vi "Measure.vi"() -> ()   [LabVIEW 2013]
uses:
  <vilib>/Utility/error.llb/DialogType.ctl
panel:
  in  "errorOutt":errorcluster
  in  "m1":string=" INSTRUCTIONS:\r\rNormal Use:  When using subVIs that incorporate the error in/error out (or error I/O) structure, place this handler where you want to inform the user of an error, typically at the end of the I/O data path, as the last action of the program.  If the error in error? is ERROR, the handler creates a message describing the error and its source.  If the type of dialog = 1 (default), the message is displayed to the user, who can only acknowedge it.  If the type = 2, the user can acknowledge the message or abort execution; aborting a program with active I/O is not recommended.  If the type = 0, no message is displayed; this is used to process the error programmatically, and the error out cluster elements are wired to individual terminals for that reason.  \r\rOther Use:\n\r\nlocal testing.  To test the error code of a subVI or function that does not have the error I/O structure, you can wire its error code and a source string to the local error code and error source inputs.  If error in error? indicates no error and error code is not equal to 0, the local code and source are substituted for the error in values, and error? is set TRUE (ERROR)."
  in  "Error":bool
  in  "SetOutput":bool
  in  "NeedToSetOutput":bool
  out "Output":string
  out "SetCurrentStr":string
  out "SetVoltageStr":string
  in  "SetVoltage":dbl format="%#.3g"
  in  "SetCurrent":dbl
  in  "NeedToSetVoltage":bool
  in  "NeedToSetCurrent":bool
  in  "Active":bool
  out "connection ID":refnum<k5>
  in  "Connect":bool
  out "GetCurrent":string
  in  "Adress":string="172.16.21.19"
  out "GetVoltage":string
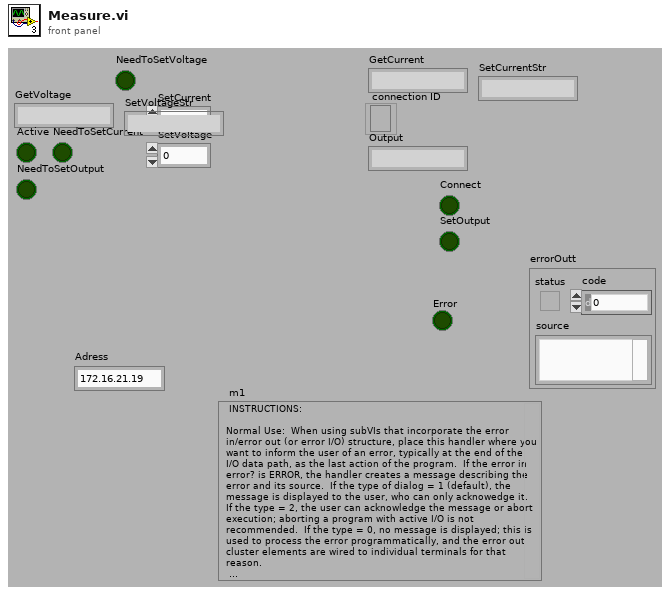
[diagram p1: front panel]
types:
  T1 = typedef "DialogType.ctl" = u16
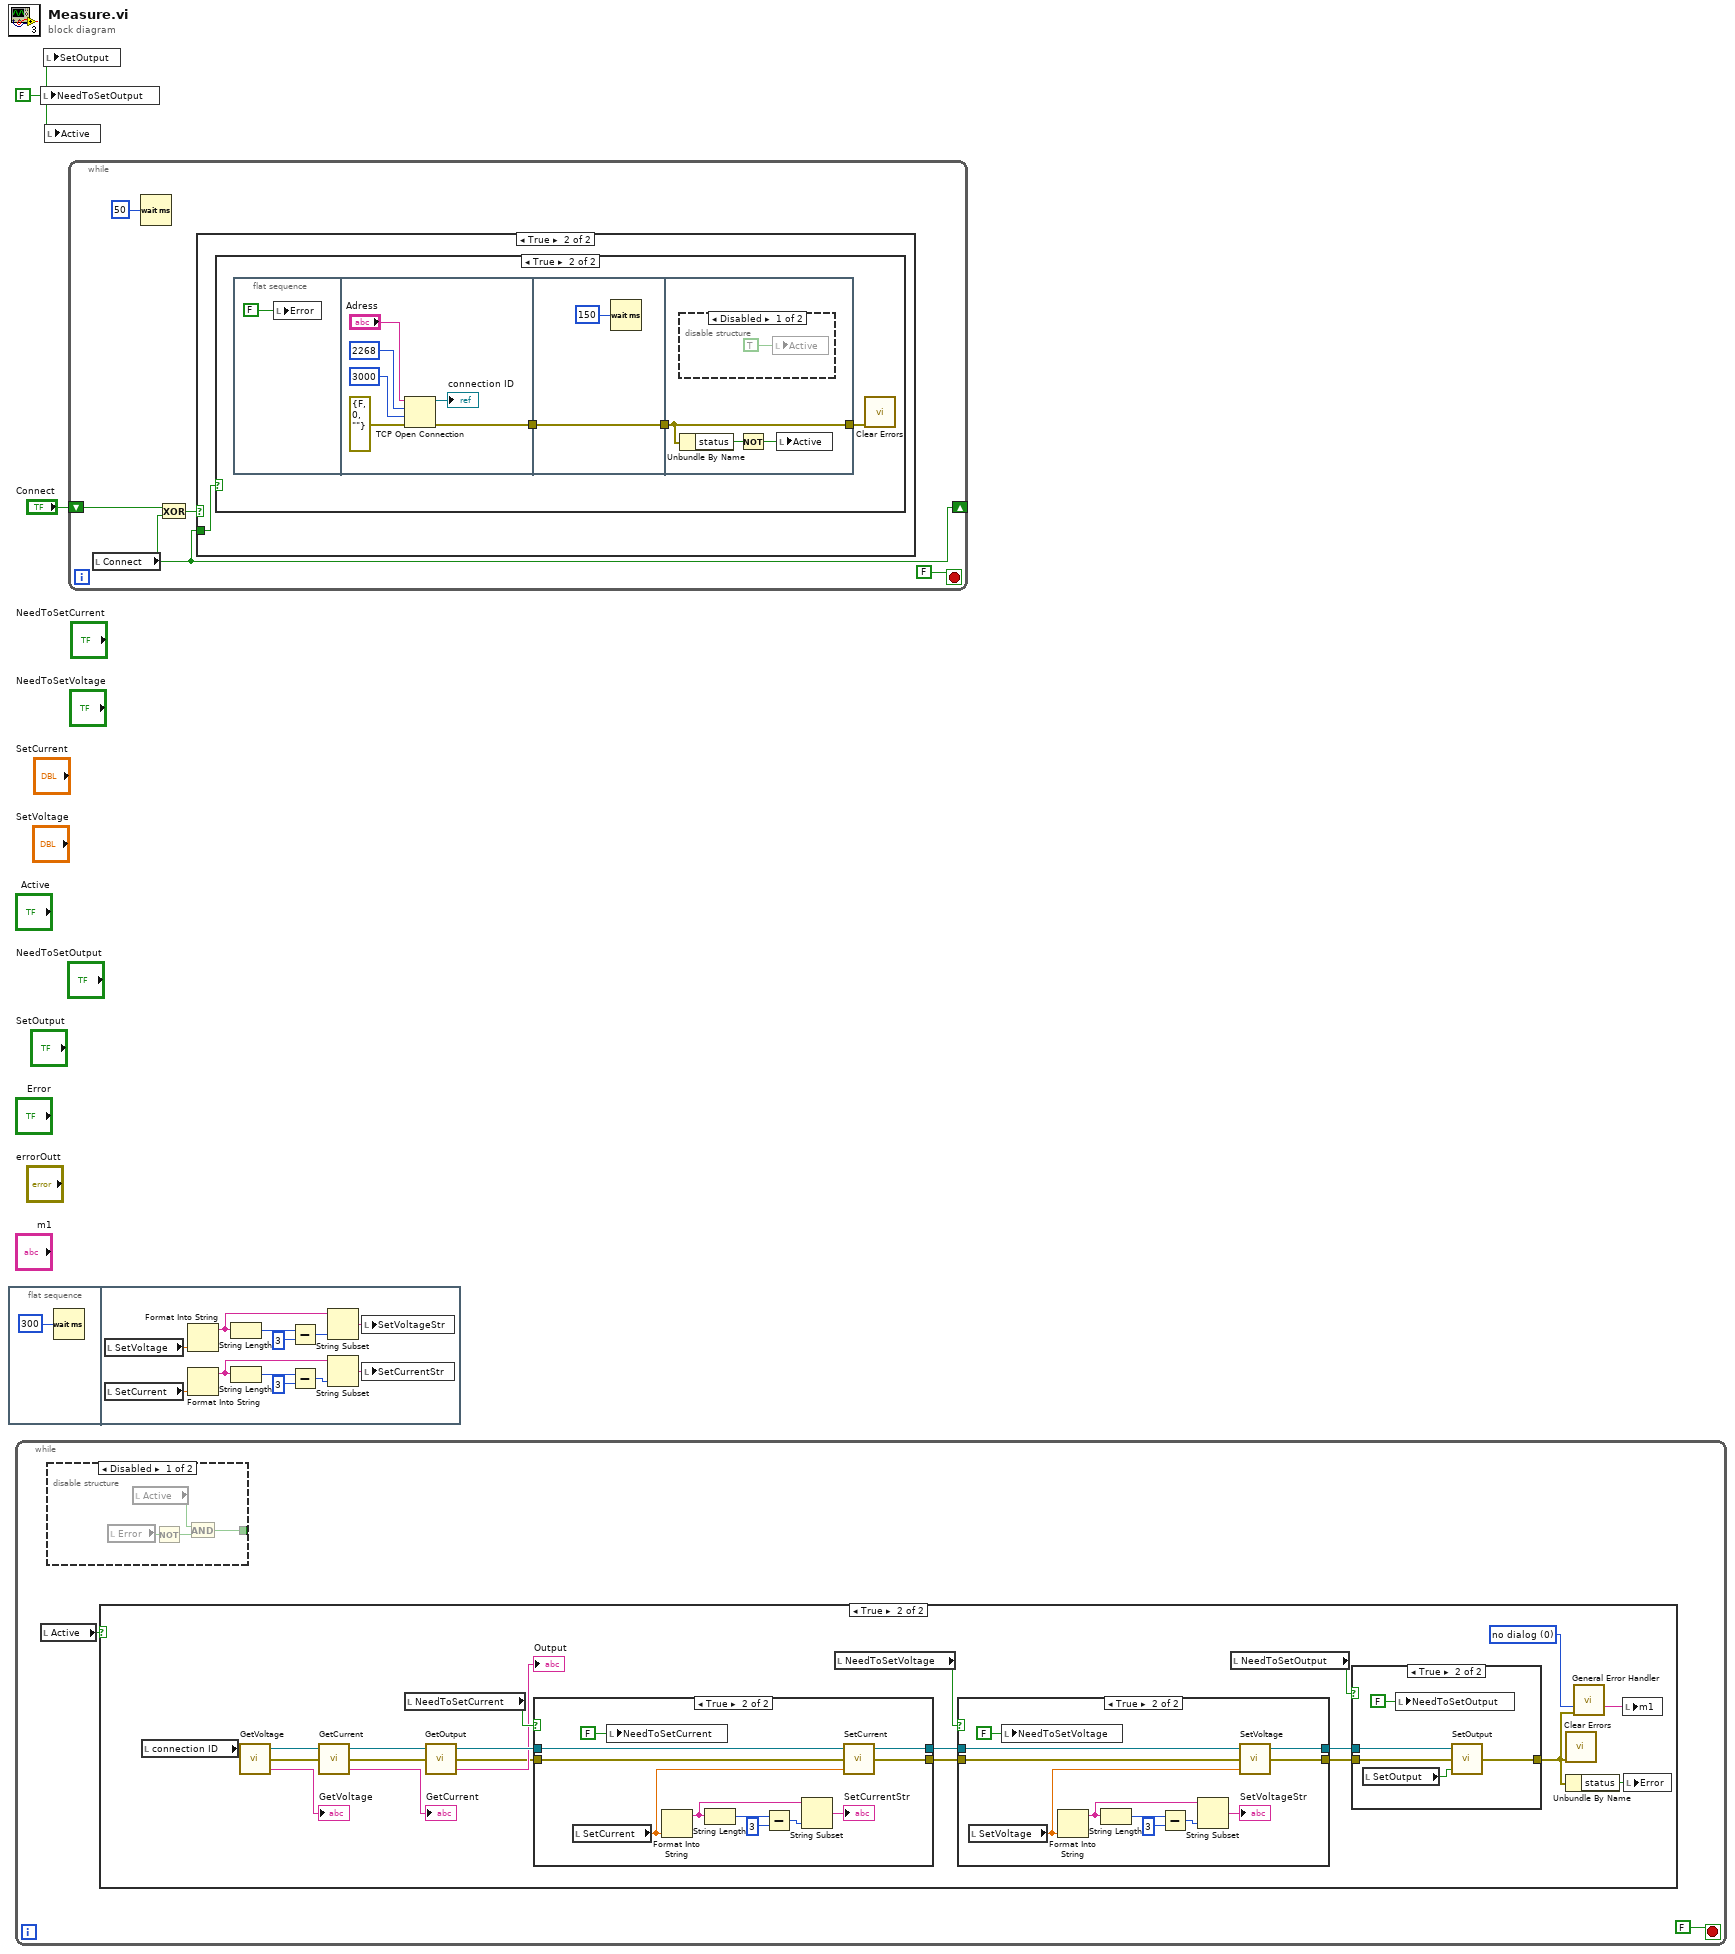
[diagram p0: block diagram]
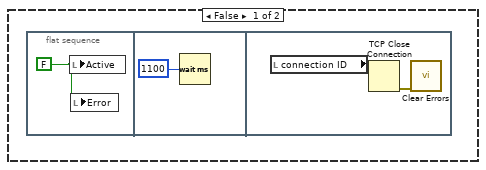
[diagram p8: hidden frame]
diagram:
  w1 = FALSE ("Active")
  n1 = flat-sequence {
    frame #0 {
      n2 = Wait (ms)(milliseconds to wait=u32 300 ("millisecond multiple")) -> ()  [unwired: 1 out]
    }
    frame #1 {
      n3 = local read "SetVoltage"() -> (w10:dbl)
      n4 = local read "SetCurrent"() -> (w11:dbl)
      n5 = Format Into String(w10) -> (resulting string=w6:string)  [unwired: 3 in, 1 out]
      n6 = Format Into String(w11) -> (resulting string=w15:string)  [unwired: 3 in, 1 out]
      n7 = String Length(string=w6) -> (length=w9:i32)
      n8 = String Length(string=w15) -> (length=w14:i32)
      n9 = Subtract(x=w9, y=3) -> (x-y=w7:i32)
      n10 = Subtract(x=w14, y=3) -> (x-y=w12:i32)
      n11 = String Subset(string=w6, length (rest)=w7) -> (substring=w5:string)  [unwired: 1 out]
      n12 = String Subset(string=w15, length (rest)=w12) -> (substring=w4:string)  [unwired: 1 out]
      n13 = local write "SetVoltageStr"(w5) -> ()
      n14 = local write "SetCurrentStr"(w4) -> ()
    }
  }
  n15 = while {
    stop <- FALSE stop-if-true
    n16 = local read "Active"() -> (w16:bool)
    n17 = disable-structure shown="Disabled" {
      disable-tunnel: [w18 _] -> _
      frame Disabled {
        n18 = local read "Error"() -> (w21:bool)
        n19 = local read "Active"() -> (w19:bool)
        n20 = Not(x=w21) -> (.not. x?=w20:bool)
        n21 = And(x=w19, y=w20) -> (x .and. y?=w18:bool)
      }
      frame Enabled {
      }
    }
    n22 = case shown="True" w16 {
      frame False {
      }
      frame True {
        w24 = T1 0 items=["no dialog", "OK message", "continue or stop message", "OK message + warnings", "continue/stop + warnings"] ("type of dialog (OK msg:1)")
        n23 = local read "connection ID"() -> (w39:refnum<k5>)
        n24 = call "GetVoltage.vi"("connection ID"=w39) -> ("Voltage"=→"GetVoltage":string, "error out"=w30:errorcluster, "connection ID out"=w41:refnum<k5>)  [unwired: 1 in, 1 out]
        n25 = call "GetCurrent.vi"("error in"=w30, "connection ID"=w41) -> ("Current"=→"GetCurrent":string, "error out"=w29:errorcluster, "connection ID out"=w35:refnum<k5>)  [unwired: 1 out]
        n26 = local read "NeedToSetCurrent"() -> (w36:bool)
        n27 = call "GetOutput.vi"("error in"=w29, "connection ID"=w35) -> ("Output"=→"Output":string, "error out"=w28:errorcluster, "connection ID out"=w34:refnum<k5>)  [unwired: 1 out]
        n28 = case shown="True" w36 {
          tunnel: w34 -> [w63 w74]
          tunnel: [w63 w73] -> w38
          tunnel: w28 -> [w62 w65]
          tunnel: [w62 w64] -> w27
          frame False {
          }
          frame True {
            n29 = local read "SetCurrent"() -> (w71:dbl)
            n30 = local write "NeedToSetCurrent"(FALSE ("NeedToSetCurrent")) -> ()
            n31 = Format Into String(w71) -> (resulting string=w66:string)  [unwired: 3 in, 1 out]
            n32 = String Length(string=w66) -> (length=w68:i32)
            n33 = Subtract(x=w68, y=3) -> (x-y=w70:i32)
            n34 = String Subset(string=w66, length (rest)=w70) -> (substring=→"SetCurrentStr":string)  [unwired: 1 out]
            n35 = call "SetCurrent.vi"("Current"=w71, "error in"=w65, "connection ID"=w74) -> ("error out"=w64:errorcluster, "connection ID out"=w73:refnum<k5>)  [unwired: 1 out]
          }
        }
        n36 = local read "NeedToSetVoltage"() -> (w37:bool)
        n37 = case shown="True" w37 {
          tunnel: w38 -> [w50 w61]
          tunnel: [w50 w53] -> w32
          tunnel: w27 -> [w49 w52]
          tunnel: [w49 w51] -> w26
          frame False {
          }
          frame True {
            n38 = local read "SetVoltage"() -> (w59:dbl)
            n39 = local write "NeedToSetVoltage"(FALSE ("NeedToSetVoltage")) -> ()
            n40 = Format Into String(w59) -> (resulting string=w55:string)  [unwired: 3 in, 1 out]
            n41 = String Length(string=w55) -> (length=w58:i32)
            n42 = Subtract(x=w58, y=3) -> (x-y=w56:i32)
            n43 = String Subset(string=w55, length (rest)=w56) -> (substring=→"SetVoltageStr":string)  [unwired: 1 out]
            n44 = call "SetVoltage.vi"("Voltage"=w59, "error in"=w52, "connection ID"=w61) -> ("error out"=w51:errorcluster, "connection ID out"=w53:refnum<k5>)  [unwired: 1 out]
          }
        }
        n45 = local read "NeedToSetOutput"() -> (w31:bool)
        n46 = case shown="True" w31 {
          tunnel: w32 -> [_ w46]
          tunnel: w26 -> [w43 w45]
          tunnel: [w43 w44] -> w22
          frame False {
          }
          frame True {
            n47 = local read "SetOutput"() -> (w47:bool)
            n48 = local write "NeedToSetOutput"(FALSE ("NeedToSetVoltage")) -> ()
            n49 = call "SetOutput.vi"("State"=w47, "error in"=w45, "connection ID"=w46) -> ("error out"=w44:errorcluster)  [unwired: 2 out]
          }
        }
        n50 = call <vilib>:"Clear Errors.vi"("error in (no error)"=w22) -> ()  [unwired: 7 out]
        n51 = Unbundle By Name(w22) -> ("status"=w25:bool)
        n52 = call <vilib>:"General Error Handler.vi"("type of dialog (OK msg:1)"=w24, "error in (no error)"=w22) -> ("message"=w23:string)  [unwired: 13 out]
        n53 = local write "m1"(w23) -> ()
        n54 = local write "Error"(w25) -> ()
      }
    }
  }
  n55 = local write "NeedToSetOutput"(w1) -> ()
  n56 = local write "SetOutput"(w1) -> ()
  n57 = local write "Active"(w1) -> ()
  n58 = while {
    shift-right: [w75] -> _
    shift-left: "Connect" -> [w76]
    stop <- FALSE stop-if-true
    n59 = local read "Connect"() -> (w75:bool)
    n60 = Wait (ms)(milliseconds to wait=u32 50 ("millisecond multiple")) -> ()  [unwired: 1 out]
    n61 = Exclusive Or(1:w75, 2:w76) -> (0:w77:bool)
    n62 = case shown="True" w77 {
      tunnel: w75 -> [_ w80]
      frame False {
      }
      frame True {
        n63 = case shown="True" w80 {
          frame False {
            n64 = flat-sequence {
              frame #0 {
                w81 = FALSE ("Active")
                n65 = local write "Active"(w81) -> ()
                n66 = local write "Error"(w81) -> ()
              }
              frame #1 {
                n67 = Wait (ms)(milliseconds to wait=u32 1100 ("millisecond multiple")) -> ()  [unwired: 1 out]
              }
              frame #2 {
                n68 = local read "connection ID"() -> (w84:refnum<k5>)
                n69 = TCP Close Connection(connection ID=w84) -> (error out=w83:errorcluster)  [unwired: 1 in, 2 out]
                n70 = call <vilib>:"Clear Errors.vi"("error in (no error)"=w83) -> ()  [unwired: 7 out]
              }
            }
          }
          frame True {
            n71 = flat-sequence {
              tunnel: [w89] -> w86
              tunnel: [w95] -> w87
              tunnel: w86 -> [w95]
              tunnel: w87 -> [w99]
              tunnel: [w99] -> w85
              frame #0 {
                n72 = local write "Error"(FALSE ("Error")) -> ()
              }
              frame #1 {
                n73 = TCP Open Connection(address="Adress", remote port or service name=u16 2268 ("Port"), timeout ms (60000)=3000, error in (no error)=errorcluster {"status"=FALSE, "code"=0, "source"=""}) -> (connection ID=→"connection ID":refnum<k5>, error out=w89:errorcluster)  [unwired: 1 out]
              }
              frame #2 {
                n74 = Wait (ms)(milliseconds to wait=u32 150 ("millisecond multiple")) -> ()  [unwired: 1 out]
              }
              frame #3 {
                n75 = disable-structure shown="Disabled" {
                  frame Disabled {
                    n76 = local write "Active"(TRUE) -> ()
                  }
                  frame Enabled {
                  }
                }
                n77 = Unbundle By Name(w99) -> ("status"=w98:bool)
                n78 = Not(x=w98) -> (.not. x?=w97:bool)
                n79 = local write "Active"(w97) -> ()
              }
            }
            n80 = call <vilib>:"Clear Errors.vi"("error in (no error)"=w85) -> ()  [unwired: 7 out]
          }
        }
      }
    }
  }
